vi "Get Property ID and Help Text from File.vi"(11 "Path":path=path "C:/Users/Quentin/Desktop/LabVIEW Help HTML/lvprop.chm/TabControl_Tab_Into.html") -> (0 "Context Help":string, 1 "ShortName":string, 2 "Class":string, 3 "Found?":bool, 4 "Available in Run-Time":string)   [LabVIEW 2015]
doc: "<b> </b> <b> </b>\n©2016 Q Software Innovations, LLC (QSI)\nwritten by Quentin Alldredge\nproduced in LabVIEW 2015"
uses:
  <vilib>/regexp/Match Regular Expression.xnode
  Q Toolbox/Q Toolbox.lvlib
panel:
  out "text":string
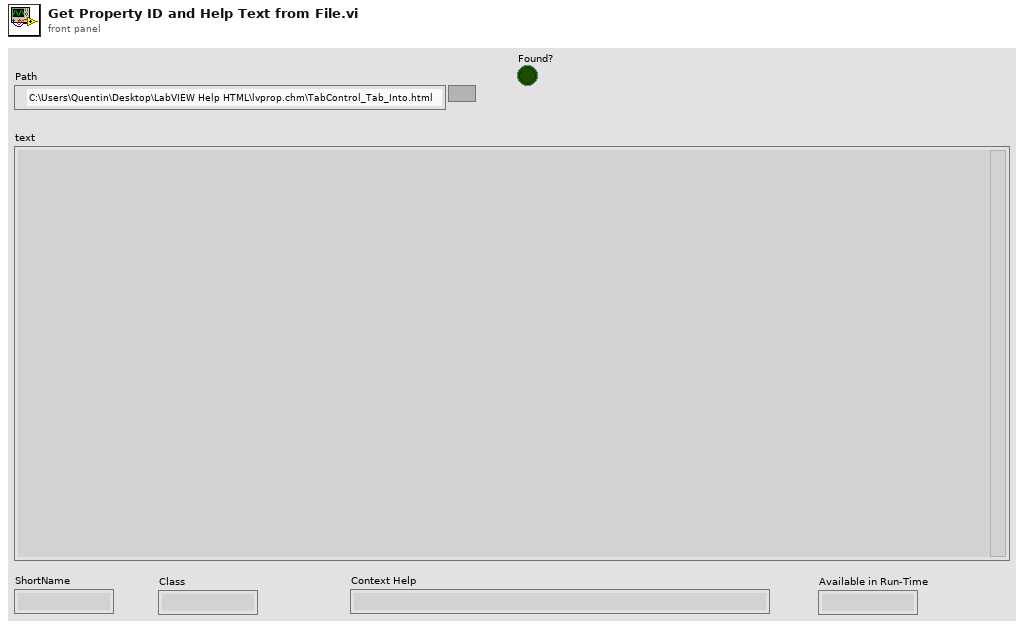
[diagram p1: front panel]
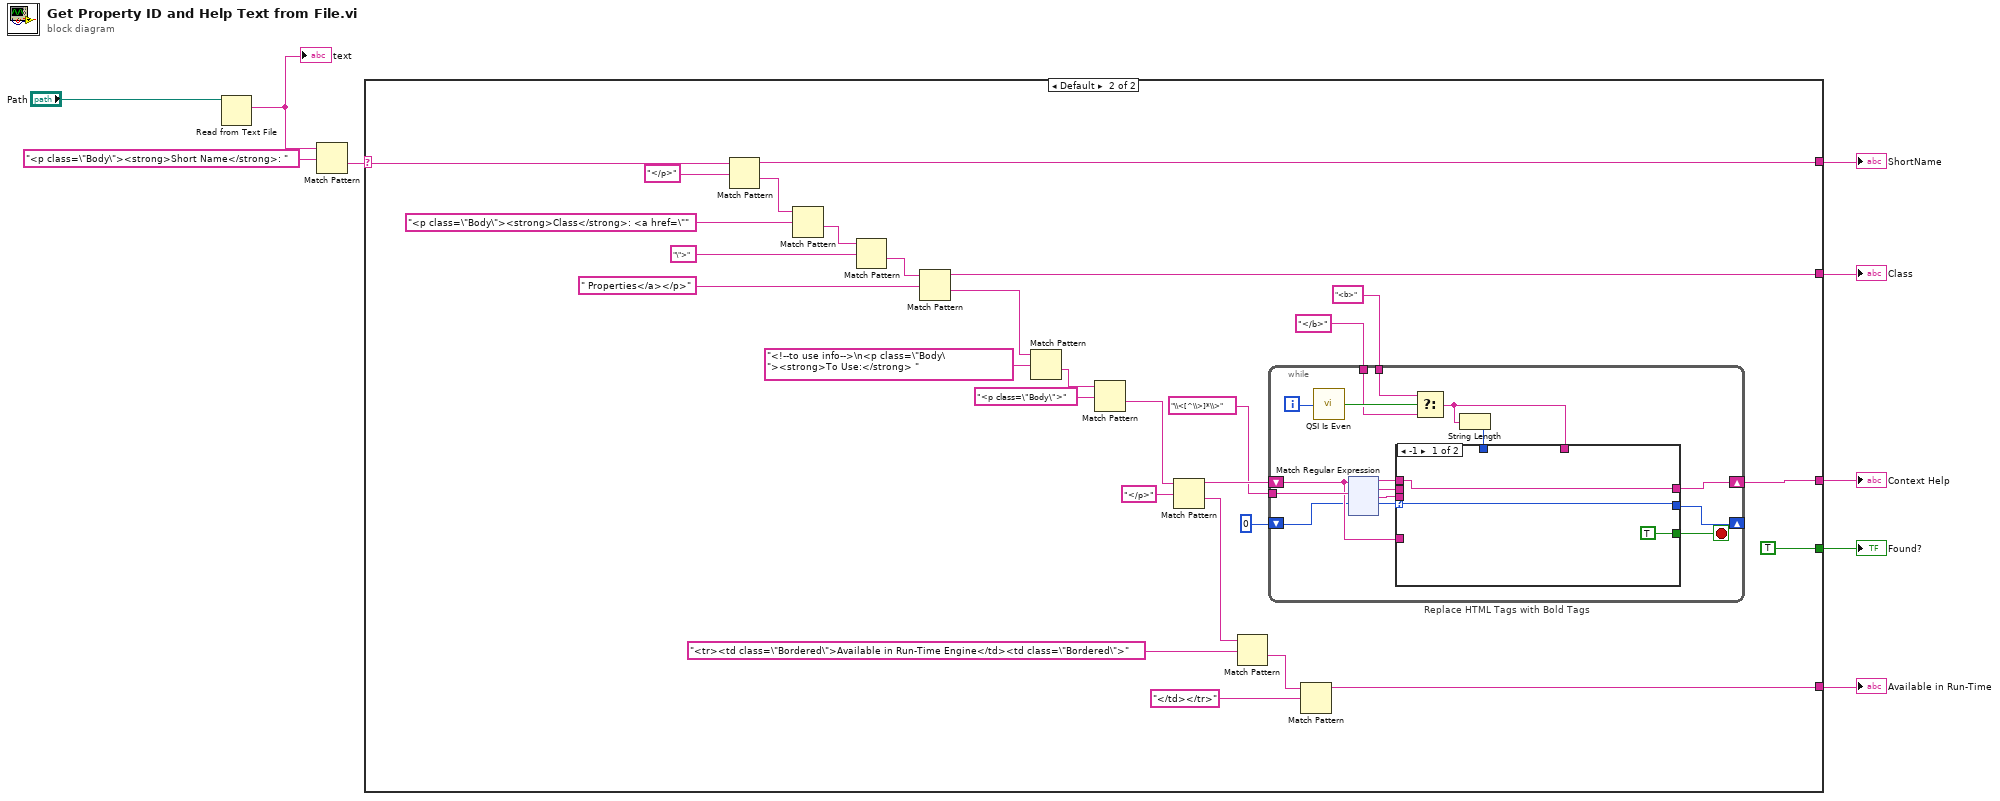
[diagram p0: block diagram]
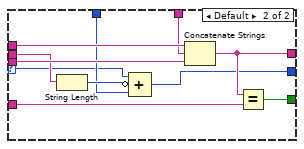
[diagram p3: hidden frame]
diagram:
  n1 = Read from Text File(file (use dialog)="Path") -> (text=w8:string)  [unwired: 3 in, 3 out]
  "text" <- w8
  n2 = Match Pattern(string=w8, regular expression="<p class=\"Body\"><strong>Short Name</strong>: ") -> (after substring=w6:string)  [unwired: 1 in, 3 out]
  n3 = case shown="Default" w6 {
    selector: w6 -> [_ w31]
    tunnel: [_ w18] -> w5
    tunnel: [_ w30] -> w4
    tunnel: [_ TRUE] -> w3
    tunnel: [_ w22] -> w2
    tunnel: [_ w10] -> w1
    frame "" {
    }
    frame Default {
      n4 = Match Pattern(string=w31, regular expression="</p>") -> (before substring=w30:string, after substring=w28:string)  [unwired: 1 in, 2 out]
      n5 = Match Pattern(string=w28, regular expression="<p class=\"Body\"><strong>Class</strong>: <a href=\"") -> (after substring=w26:string)  [unwired: 1 in, 3 out]
      n6 = Match Pattern(string=w26, regular expression="\">") -> (after substring=w24:string)  [unwired: 1 in, 3 out]
      n7 = Match Pattern(string=w24, regular expression=" Properties</a></p>") -> (before substring=w22:string, after substring=w21:string)  [unwired: 1 in, 2 out]
      n8 = Match Pattern(string=w21, regular expression="<!--to use info-->\n<p class=\"Body\"><strong>To Use:</strong> ") -> (after substring=w36:string)  [unwired: 1 in, 3 out]
      n9 = Match Pattern(string=w36, regular expression="<p class=\"Body\">") -> (after substring=w33:string)  [unwired: 1 in, 3 out]
      n10 = Match Pattern(string=w33, regular expression="</p>") -> (before substring=w20:string, after substring=w14:string)  [unwired: 1 in, 2 out]
      n11 = Match Pattern(string=w14, regular expression="<tr><td class=\"Bordered\">Available in Run-Time Engine</td><td class=\"Bordered\">") -> (after substring=w12:string)  [unwired: 1 in, 3 out]
      n12 = while "Replace HTML Tags with Bold Tags" {
        tunnel: "\\<[^\\>]*\\>" ("regular expression") -> [w53]
        shift-right: [w49] -> w18
        shift-left: w20 -> [w50]
        tunnel: "<b>" ("regular expression") -> [w44]
        tunnel: "</b>" ("regular expression") -> [w43]
        shift-right: [w38] -> _
        shift-left: 0 -> [w47]
        i -> [w46]
        stop <- w48 stop-if-true
        n13 = call "QSI Is Even.vi"("Number"=w46) -> ("Is Even?"=w45:bool)  [unwired: 4 in]
        n14 = xnode "Match Regular Expression"("input string"=w50, "regular expression"=w53, "offset (0)"=w47) -> ("before match"=w52:string, "whole match"=w42:string, "after match"=w51:string, "offset past match"=w39:i32)  [unwired: 3 in, 1 out]
        n15 = Select(t=w44, s=w45, f=w43) -> (s? t:f=w41:string)
        n16 = String Length(string=w41) -> (length=w40:i32)
        n17 = case shown="-1" w39 {
          selector: w39 -> [w55 w58]
          tunnel: w52 -> [w56 w67]
          tunnel: w51 -> [_ w66]
          tunnel: w50 -> [_ w65]
          tunnel: [w56 w64] -> w49
          tunnel: [TRUE w63] -> w48
          tunnel: w42 -> [_ w62]
          tunnel: w41 -> [_ w60]
          tunnel: w40 -> [_ w59]
          tunnel: [w55 w57] -> w38
          frame -1 {
          }
          frame Default {
            n18 = String Length(string=w62) -> (length=w61:i32)
            n19 = Compound Arithmetic op=ADD(w58, invert w61, w59) -> (w57:i32)
            n20 = Concatenate Strings(w67, w60, w66) -> (w64:string)
            n21 = Equal?(x=w64, y=w65) -> (x = y?=w63:bool)
          }
        }
      }
      n22 = Match Pattern(string=w12, regular expression="</td></tr>") -> (before substring=w10:string)  [unwired: 1 in, 3 out]
    }
  }
  "Context Help" <- w5
  "ShortName" <- w4
  "Found?" <- w3
  "Class" <- w2
  "Available in Run-Time" <- w1
